vi "Do.vi"(8 "error in":errorcluster, 10 "Actor in":refnum<class "Actor.lvclass">, 11 "Set f0 MSG":refnum<class "Set TEC SP MSG.lvclass">) -> (0 "error out":errorcluster, 2 "Actor out":refnum<class "Actor.lvclass">)   [LabVIEW 2014, in "Set TEC SP MSG.lvclass"]
doc: "(<B>Filename</B>: Actor Framework.lvlib:Message.lvclass:Do.vi)\n\nDefines what a message does when it is received by an actor. Generally, a message instructs an actor to invoke one of its methods. By default, this method does nothing. A child class must override it to define behavior. Create a child class by using the Actor Framework Message Maker dialog box."
uses:
  Set TEC SP MSG.lvclass
  <vilib>/ActorFramework/Actor/Actor.lvclass
  Set TEC SP MSG.lvclass/Set TEC SP MSG.ctl
  Instr Actor.lvclass
  PAS/Commands/Change TEC SPs/Change TEC SPs.lvclass
  PAS/Commands/Change TEC SPs/Change TEC SPs.lvclass/Change TEC SPs.ctl
  Controller/Messages/Update Settings/Children/Array Data/SGL/Update SGL Array.lvclass
  Controller/Messages/Update Settings/Update Setting.lvclass/Update Setting.ctl
  Controller/Messages/Update Settings/Children/Array Data/SGL/Update SGL Array.lvclass/Update SGL Array.ctl
  Controller/Messages/Update Settings/Write Key.vi
  Controller/Messages/Update Settings/Children/Array Data/SGL/Write Setting.vi
  PAS/Commands/Change TEC SPs/Write SP.vi
  reusable/Command/Command.lvclass
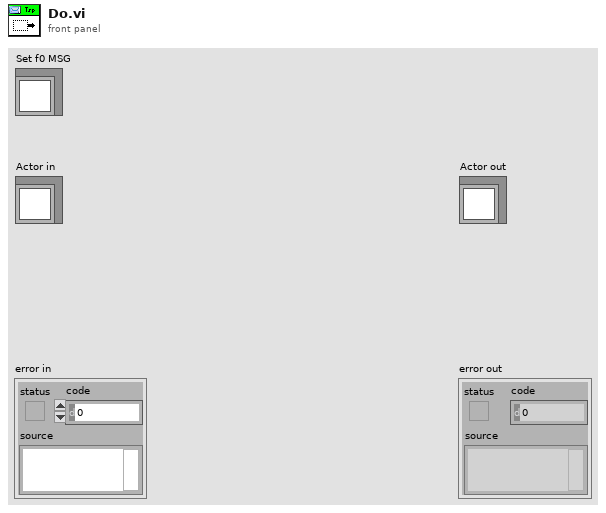
[diagram p1: front panel]
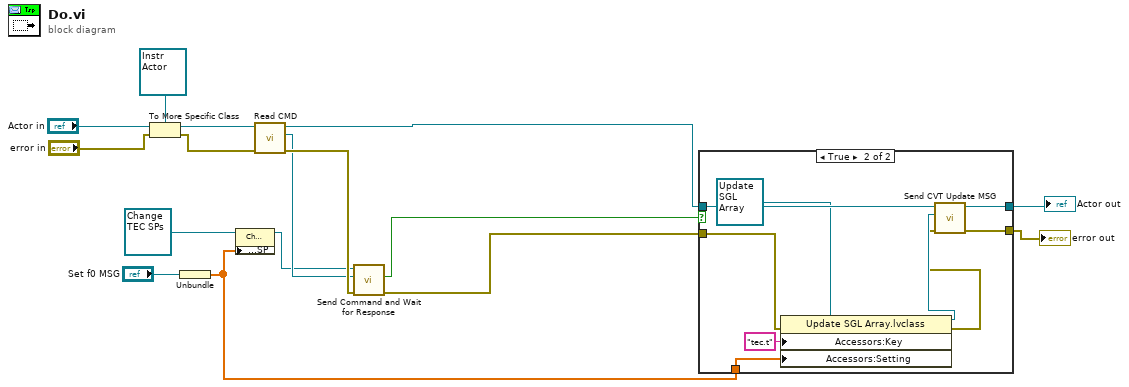
[diagram p0: block diagram]
diagram:
  n1 = To More Specific Class(target class=refnum<class "Instr Actor.lvclass"> refnum ("Instrument Lib:Instr"), reference="Actor in", error in="error in") -> (specific class reference=w14:refnum<class "Instr Actor.lvclass">, error out=w13:errorcluster)
  n2 = Unbundle("Set f0 MSG") -> (w1:sgl[])
  n3 = property class="Change TEC SPs.lvclass"(reference=refnum<class "Change TEC SPs.lvclass"> refnum ("Change TEC SPs.lvclass"), "Accessors:SP"=w1) -> (reference out=w7:refnum<class "Change TEC SPs.lvclass">)  [unwired: 1 in, 1 out]
  n4 = call "Read CMD.vi"("error in (no error)"=w13, "Instr Actor in"=w14) -> ("error out"=w10:errorcluster, "CMD"=w8:refnum<queue>, "Instr Actor out"=w6:refnum<class "Instr Actor.lvclass">)  [unwired: 7 in]
  n5 = call "Send Command and Wait for Response.vi"("error in"=w10, "cmd queue"=w8, "CMD in"=w7) -> ("error out"=w2:errorcluster, "cmd good?"=w5:bool)  [unwired: 6 in, 1 out]
  n6 = case shown="True" w5 {
    tunnel: w1 -> [_ w23]
    tunnel: w6 -> [w18 w27]
    tunnel: [w18 w26] -> w3
    tunnel: w2 -> [w17 w21]
    tunnel: [w17 w25] -> w4
    frame False {
    }
    frame True {
      n7 = property class="Update SGL Array.lvclass"(reference=refnum<class "Update SGL Array.lvclass"> refnum ("Controller.lvlib:Update SGL Array.lvclass"), error in=w21, "Accessors:Key"="tec.t" ("Key"), "Accessors:Setting"=w23) -> (reference out=w22:refnum<class "Update SGL Array.lvclass">, error out=w20:errorcluster)
      n8 = call "Send CVT Update MSG.vi"("error in (no error)"=w20, "Update Setting"=w22, "Instr in"=w27) -> ("error out"=w25:errorcluster, "Instr out"=w26:refnum<class "Instr Actor.lvclass">)  [unwired: 7 in]
    }
  }
  "error out" <- w4
  "Actor out" <- w3
